vi "ForLoopCh2.vi"() -> ()   [LabVIEW 2017]
panel:
  out "Array":dbl[](array[numeric])
  out "Waveform Graph":cluster{"y":dbl, "y":dbl, dbl[]}(graph)
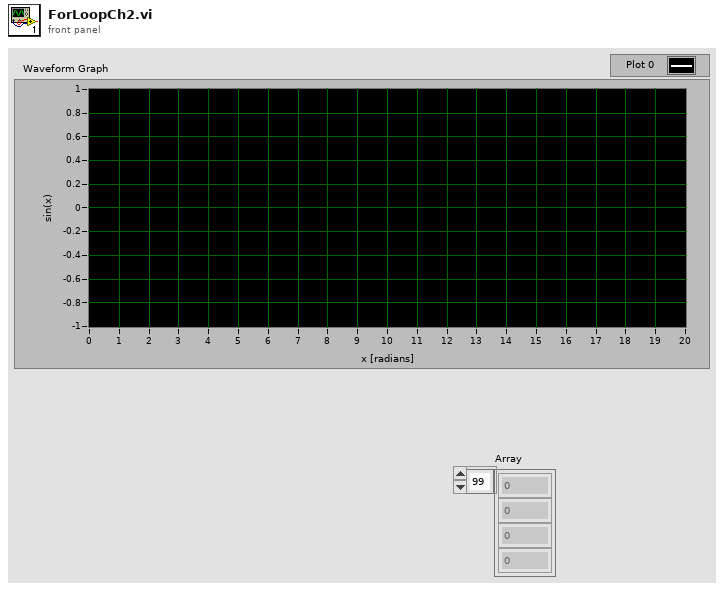
[diagram p1: front panel]
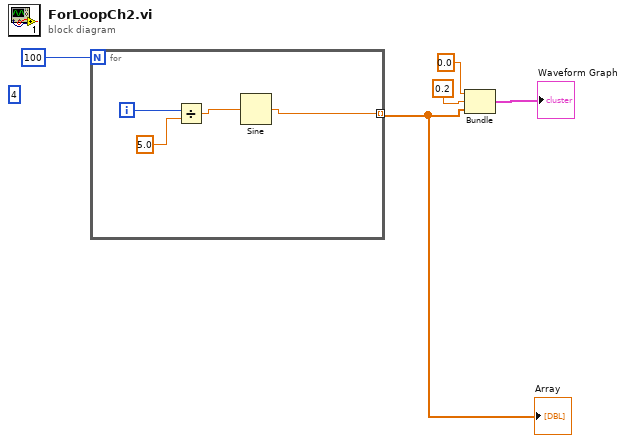
[diagram p0: block diagram]
diagram:
  (unwired) 4 ("y")
  n1 = for {
    N: 100 -> [_]
    tunnel: [w6] -> w1 mode=indexing
    i -> [w9]
    n2 = Divide(x=w9, y=5.0) -> (x/y=w7:dbl)
    n3 = Sine(x=w7) -> (sin(x)=w6:dbl)
  }
  "Array" <- w1
  n4 = Bundle("y"=0.0, "y"=0.2, w1) -> (→"Waveform Graph":cluster{"y":dbl, "y":dbl, dbl[]})  [unwired: 1 in]
